vi "Next Step.vi"(8 "error in (no error)":errorcluster, 11 "Continuous.lvclass in":refnum<class "Continuous.lvclass">) -> (0 "error out":errorcluster, 1 "Step #":u32, 2 "actual position":dbl, 3 "Continuous.lvclass out":refnum<class "Continuous.lvclass">)   [LabVIEW 2017, in "Continuous.lvclass"]
uses:
  Continuous.lvclass
  Instruments/Oxford Magnet/Power Supply/Power Supply.lvclass
  C:/LabVIEW-programs/Instruments/Utility Classes/Scannable/Scannable.lvclass
  Scanner/Scanner.lvclass
panel:
  in  "Manual Override":bool
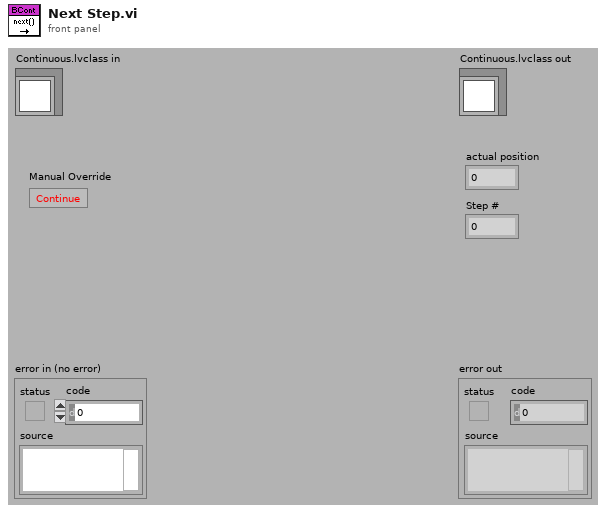
[diagram p1: front panel]
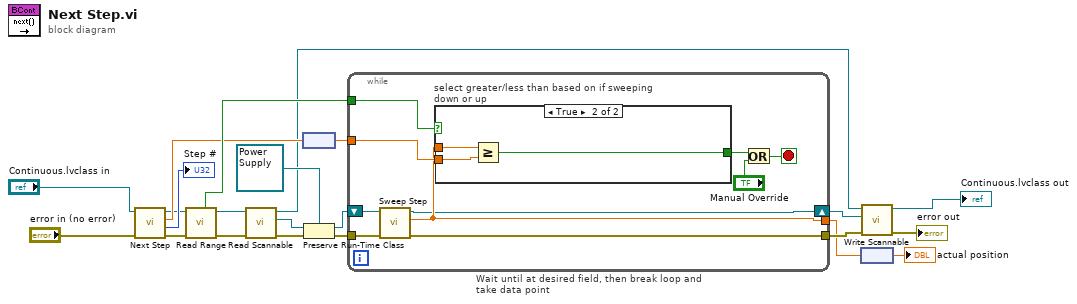
[diagram p0: block diagram]
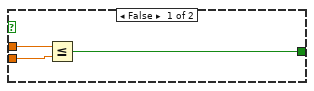
[diagram p2: hidden frame]
diagram:
  n1 = call-parent "Next Step.vi"("error in (no error)"="error in (no error)", "Scanner in"="Continuous.lvclass in") -> ("error out"=w18:errorcluster, "Current Step"=→"Step #":u32, "Current Position"=w19:dbl, "Scanner out"=w16:refnum<class "Continuous.lvclass">)  [unwired: 6 out]
  n2 = call-dynamic "Read Range.vi"("error in (no error)"=w18, "Scanner.lvclass in"=w16) -> ("error out"=w7:errorcluster, "Scanner.lvclass out"=w6:refnum<class "Continuous.lvclass">, "Scanning Up?"=w21:bool)  [unwired: 7 out]
  n3 = call-dynamic "Read Scannable.vi"("error in (no error)"=w7, "Scanner.lvclass in"=w6) -> ("error out"=w14:errorcluster, "Scannable.lvclass"=w13:refnum<class "Scannable.lvclass">, "Scanner.lvclass out"=w5:refnum<class "Continuous.lvclass">)  [unwired: 7 in]
  n4 = node(w19) -> (w15:dbl[unit])
  n5 = Preserve Run-Time Class(object in=w13, error in=w14, 2:refnum<class "Power Supply.lvclass"> refnum ("Power Supply in")) -> (object out=w11:refnum<class "Power Supply.lvclass">, error out=w8:errorcluster)
  n6 = while "Wait until at desired field, then break loop and take data point" {
    tunnel: [w31] -> w2
    tunnel: w15 -> [w32]
    tunnel: w21 -> [w30]
    shift-right: [w25] -> w10
    shift-left: w11 -> [w26]
    tunnel: [w24] -> w9
    tunnel: w8 -> [w23]
    stop <- w29 stop-if-true
    n7 = call-dynamic "Sweep Step.vi"("error in (no error)"=w23, "Power Supply in"=w26) -> ("error out"=w24:errorcluster, "field"=w31:dbl[unit], "Power Supply out"=w25:refnum<class "Power Supply.lvclass">)  [unwired: 5 in, 2 out]
    n8 = case "select greater/less than based on if sweeping down or up" shown="True" w30 {
      tunnel: w31 -> [w34 w38]
      tunnel: w32 -> [w35 w37]
      tunnel: [w33 w36] -> w28
      frame False {
        n9 = Less Or Equal?(x=w34, y=w35) -> (x <= y?=w33:bool)
      }
      frame True {
        n10 = Greater Or Equal?(x=w38, y=w37) -> (x >= y?=w36:bool)
      }
    }
    n11 = Or(x=w28, y="Manual Override") -> (x .or. y?=w29:bool)
  }
  n12 = node(w2) -> (→"actual position":dbl)
  n13 = call-dynamic "Write Scannable.vi"("error in (no error)"=w9, "Scannable.lvclass"=w10, "Scanner.lvclass in"=w5) -> ("error out"=→"error out":errorcluster, "Scanner.lvclass out"=→"Continuous.lvclass out":refnum<class "Continuous.lvclass">)  [unwired: 7 in]
